vi "Global_info.vi"() -> ()   [LabVIEW 2015]
panel:
  in  "Cluster":T1
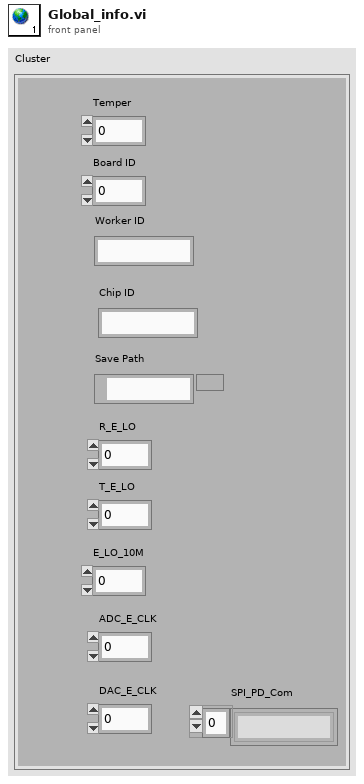
[diagram p1: front panel]
types:
  T1 = cluster{"Temper":dbl, "Board ID":u32, "Worker ID":string, "Chip ID":string, "Save Path":path, "R_E_LO":dbl, "T_E_LO":dbl, "E_LO_10M":dbl, "ADC_E_CLK":dbl, "DAC_E_CLK":dbl, "SPI_PD_Com":string[]}
diagram:
